vi "SetTstDist.vi"(6 "错误输入（无错误）":errorcluster, 8 "检测范围":sgl) -> (0 "错误输出":errorcluster)   [LabVIEW 2018]
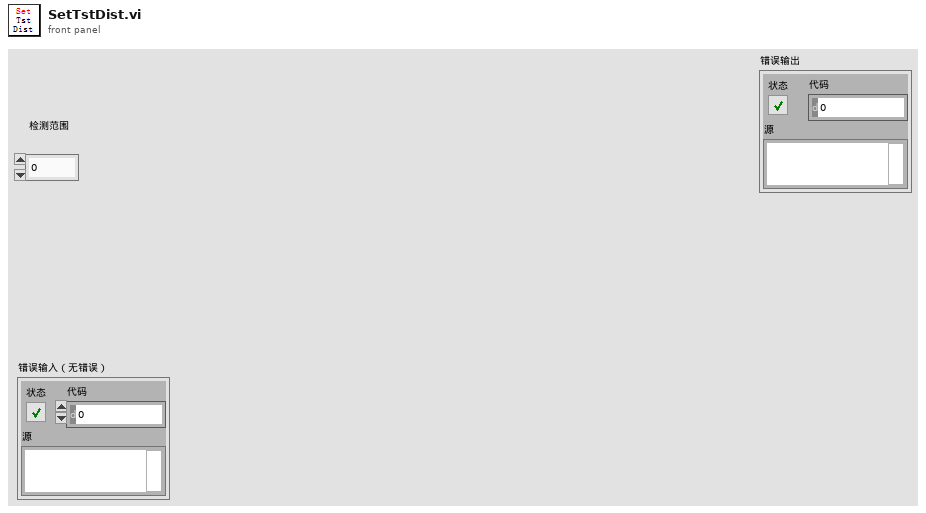
[diagram p1: front panel]
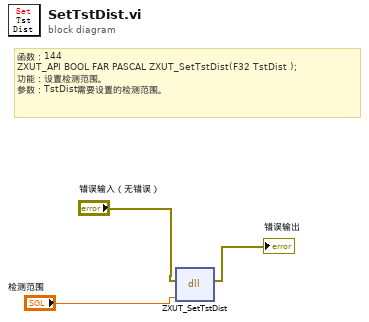
[diagram p0: block diagram]
diagram:
  # "函数：144\nZXUT_API BOOL\tFAR PASCAL ZXUT_SetTstDist(F32 TstDist );\n功能：设置检测范围。\n参数：TstDist需要设置的检测范围。"
  n1 = dll-call lib="PTH2Rabs E软件项目超声超声子VI函数VI\tTCG处理ZXUTConfigMgr.dll" fn="ZXUT_SetTstDist"(error in="错误输入（无错误）", "TstDis"="检测范围") -> (error out=→"错误输出":errorcluster)  [unwired: 4 in, 1 out]
